vi "ITC503_Temp_Readout_DP_ver1.0.vi"(0 "GPIB ADR (18)":i16=18, 1 "Enable ChD (F)":bool, 7 "Mode: (default: 2)":i16(ring)=2 items=["Do nothing to mark the end of the transfer", "Send NL (linefeed) with EOI after the data bytes.", "Send EOI with the last data byte in the string(default)"], 11 "error in":errorcluster) -> (2 "Sensor A (K)":dbl format="%.3f", 3 "Sensor A (K)":string, 4 "dump GPIB ADR":i16, 6 "Sensor B (K)":dbl format="%.3f", 8 "Sensor B (K)":string, 10 "Sensor C (K)":dbl format="%.3f", 12 "Sensor D (K)":dbl format="%.3f", 13 "Sensor D (K)":string, 14 "error out":errorcluster, 15 "Sensor C (K)":string)   [LabVIEW 2011]
doc: "This returns the field in the sample chamber as reported by the PPMS system. Note that this is not the exact field, only that calculated from the current through the magnet."
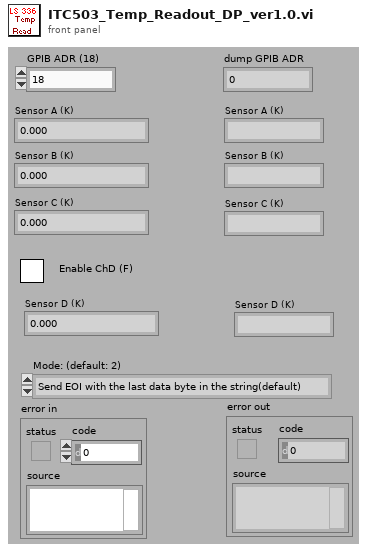
[diagram p1: front panel]
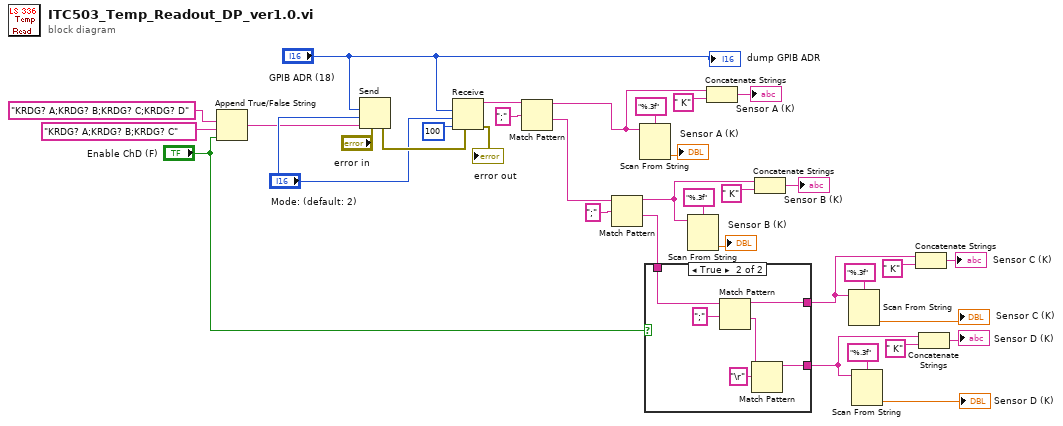
[diagram p0: block diagram]
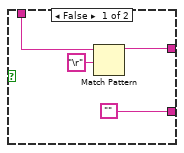
[diagram p2: hidden frame]
diagram:
  n1 = Append True/False String(1:"Enable ChD (F)", 2:"KRDG? A;KRDG? B;KRDG? C", 3:"KRDG? A;KRDG? B;KRDG? C;KRDG? D") -> (0:w9:string)  [unwired: 1 out]
  n2 = Send(2:"GPIB ADR (18)", 3:"Mode: (default: 2)", 4:"error in", 5:w9) -> (8:w25:errorcluster)  [unwired: 1 in, 2 out]
  n3 = Receive(4:w25, 6:100, 7:"Mode: (default: 2)", 8:"GPIB ADR (18)") -> (0:→"error out":errorcluster, 3:w27:string)  [unwired: 1 in, 2 out]
  n4 = Match Pattern(string=w27, regular expression=";") -> (before substring=w23:string, after substring=w21:string)  [unwired: 3 out]
  n5 = Match Pattern(string=w21, regular expression=";") -> (before substring=w16:string, after substring=w4:string)  [unwired: 3 out]
  n6 = Scan From String(format string="%.3f", input string=w23) -> (output 1=→"Sensor A (K)":dbl)  [unwired: 2 in, 4 out]
  n7 = case shown="True" "Enable ChD (F)" {
    tunnel: w4 -> [w37 w44]
    tunnel: [w38 w41] -> w2
    tunnel: ["" w40] -> w1
    frame False {
      n8 = Match Pattern(string=w37, regular expression="\r") -> (before substring=w38:string)  [unwired: 4 out]
    }
    frame True {
      n9 = Match Pattern(string=w44, regular expression=";") -> (before substring=w41:string, after substring=w43:string)  [unwired: 3 out]
      n10 = Match Pattern(string=w43, regular expression="\r") -> (before substring=w40:string)  [unwired: 4 out]
    }
  }
  n11 = Scan From String(format string="%.3f", input string=w16) -> (output 1=→"Sensor B (K)":dbl)  [unwired: 2 in, 4 out]
  n12 = Concatenate Strings(w23, " K" ("string")) -> (→"Sensor A (K)":string)
  n13 = Concatenate Strings(w16, " K" ("string")) -> (→"Sensor B (K)":string)
  n14 = Scan From String(format string="%.3f", input string=w2) -> (output 1=→"Sensor C (K)":dbl)  [unwired: 2 in, 4 out]
  n15 = Scan From String(format string="%.3f", input string=w1) -> (output 1=→"Sensor D (K)":dbl)  [unwired: 2 in, 4 out]
  n16 = Concatenate Strings(w2, " K" ("string")) -> (→"Sensor C (K)":string)
  n17 = Concatenate Strings(w1, " K" ("string")) -> (→"Sensor D (K)":string)
  "dump GPIB ADR" <- "GPIB ADR (18)"
